vi "Build Channel Group Info.vi"(8 "Channel Data Reference":i32, 9 "Channel Groups in":T2(array[cluster]), 10 "Group Name":string, 11 "Channel Type":T1=enum."Input/Read") -> (1 "Channel Groups out":T2(array[cluster]))   [LabVIEW 2026, in "Template Deployment Hooks.lvlib"]
uses:
  Template Deployment Hooks.lvlib
  Types/Channel Mode.ctl
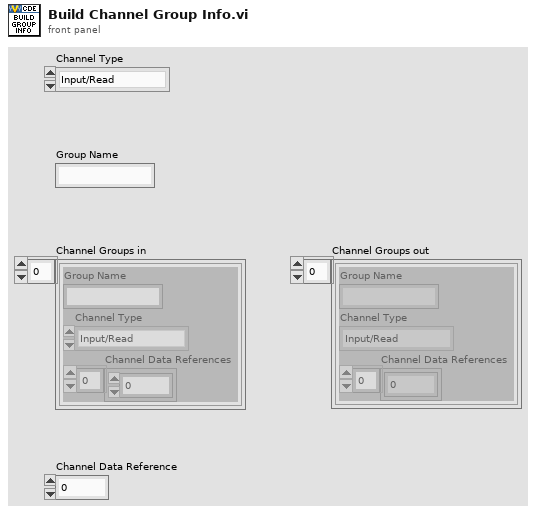
[diagram p1: front panel]
types:
  T1 = typedef "Template Deployment Hooks.lvlib/Channel Mode.ctl" = enum16{"Output/Write", "Input/Read", "Input/ReadWrite"}
  T2 = cluster{"Group Name":string, "Channel Type":T1, "Channel Data References":i32[]}[]
  T3 = cluster{"Group Name":string, "Channel Type":T1, i32[]}
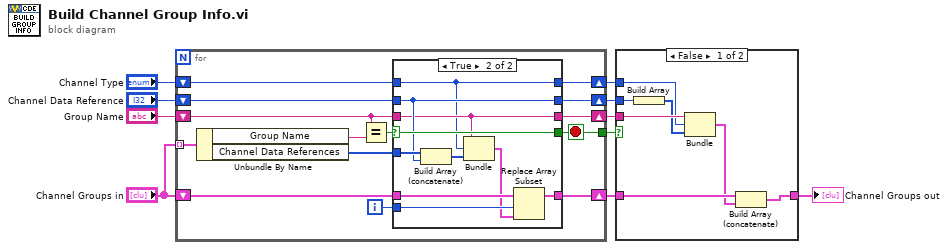
[diagram p0: block diagram]
diagram:
  n1 = for {
    tunnel: "Channel Groups in" -> [w24] mode=indexing
    shift-right: [w17] -> w7
    shift-left: "Channel Groups in" -> [w22]
    tunnel: [w15] -> w6
    shift-right: [w14] -> w10
    shift-left: "Channel Data Reference" -> [w20]
    shift-right: [w13] -> w9
    shift-left: "Group Name" -> [w18]
    shift-right: [w11] -> w1
    shift-left: "Channel Type" -> [w12]
    i -> [w19]
    stop <- w15 stop-if-true
    n2 = Unbundle By Name(w24) -> ("Group Name"=w23:string, "Channel Data References"=w21:i32[])
    n3 = Equal?(x=w18, y=w23) -> (x = y?=w16:bool)
    n4 = case shown="True" w16 {
      selector: w16 -> [w28 w34]
      tunnel: w22 -> [w29 w38]
      tunnel: w21 -> [_ w39]
      tunnel: w20 -> [w27 w33]
      tunnel: w19 -> [_ w37]
      tunnel: w18 -> [w26 w32]
      tunnel: [w29 w35] -> w17
      tunnel: [w28 w34] -> w15
      tunnel: [w27 w33] -> w14
      tunnel: [w26 w32] -> w13
      tunnel: w12 -> [w25 w31]
      tunnel: [w25 w31] -> w11
      frame False {
      }
      frame True {
        n5 = Build Array (concatenate)(w39, w33) -> (w30:i32[])
        n6 = Bundle("Group Name"=w32, "Channel Type"=w31, w30) -> (w36:T3)  [unwired: 1 in]
        n7 = Replace Array Subset(array=w38, new element=w36, index=w37) -> (w35:T2)
      }
    }
  }
  n8 = case shown="False" w6 {
    tunnel: w7 -> [w46 w47]
    tunnel: [w42 w47] -> w8
    tunnel: w9 -> [w45 _]
    tunnel: w10 -> [w44 _]
    tunnel: w1 -> [w41 _]
    frame False {
      n9 = Build Array(w44) -> (w40:i32[])
      n10 = Bundle("Group Name"=w45, "Channel Type"=w41, w40) -> (w43:T3)  [unwired: 1 in]
      n11 = Build Array (concatenate)(w46, w43) -> (w42:T2)
    }
    frame True {
    }
  }
  "Channel Groups out" <- w8
